vi "Build_Asylum_WriteString.vi"(8 "error in (no error)":errorcluster, 10 "valueString":string, 11 "parameterName":string) -> (0 "error out":errorcluster, 3 "String":string)   [LabVIEW 2016]
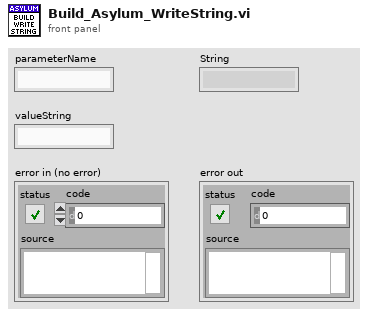
[diagram p1: front panel]
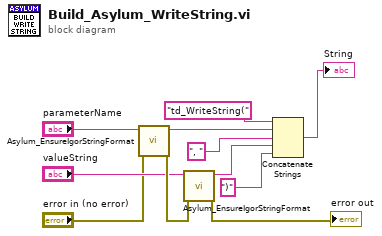
[diagram p0: block diagram]
diagram:
  n1 = call "Asylum_EnsureIgorStringFormat.vi"("error in (no error)"="error in (no error)", "Value"="parameterName") -> ("error out"=w9:errorcluster, "Value"=w5:string)  [unwired: 8 in]
  n2 = call "Asylum_EnsureIgorStringFormat.vi"("error in (no error)"=w9, "Value"="valueString") -> ("error out"=→"error out":errorcluster, "Value"=w11:string)  [unwired: 8 in]
  n3 = Concatenate Strings("td_WriteString(", w5, ", ", w11, ")" ("string")) -> (→"String":string)
